vi "IMAQ Name Create.vi"(8 "error in (no error)":errorcluster, 10 "Name (\"\")":string, 11 "Video Processor in":refnum<class "Video Processor.lvclass">) -> (0 "error out":errorcluster, 2 "Name Out":string, 3 "Video Processor out":refnum<class "Video Processor.lvclass">)   [LabVIEW 2018, in "Video Processor.lvclass"]
uses:
  Video Processor.lvclass
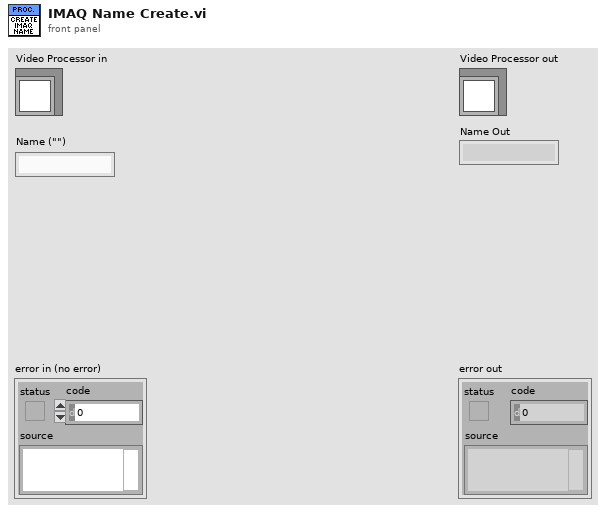
[diagram p1: front panel]
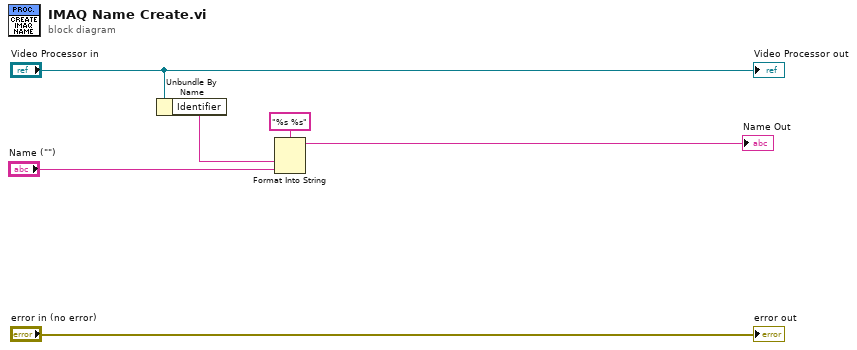
[diagram p0: block diagram]
diagram:
  n1 = Unbundle By Name("Video Processor in") -> ("Identifier"=w1:string)
  n2 = Format Into String(format string="%s %s", w1, "Name (\"\")") -> (resulting string=→"Name Out":string)  [unwired: 2 in, 1 out]
  "error out" <- "error in (no error)"
  "Video Processor out" <- "Video Processor in"
